vi "getSub2dArray.vi"(9 "Idx of Raw 1":i32[](array[numeric]), 10 "Idx of Raw 0":i32[](array[numeric]), 11 "2D Array":dbl[][](array[numeric])) -> (3 "Sub-Array":dbl[][](array[numeric]))   [LabVIEW 2016]
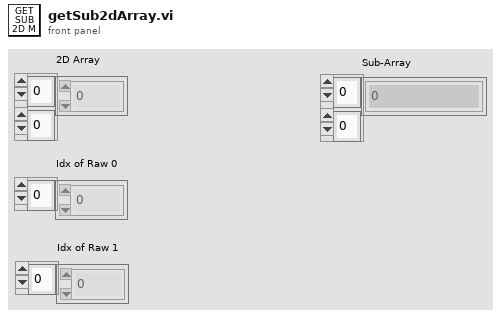
[diagram p1: front panel]
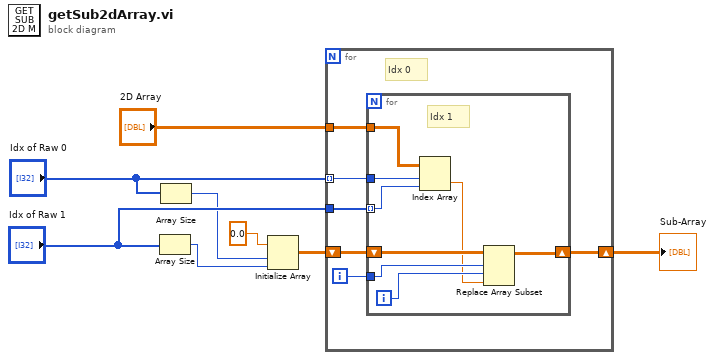
[diagram p0: block diagram]
diagram:
  n1 = Array Size(array="Idx of Raw 1") -> (size(s)=w2:i32)
  n2 = Array Size(array="Idx of Raw 0") -> (size(s)=w3:i32)
  n3 = Initialize Array(0.0 ("element"), w3, w2) -> (w6:dbl[][])
  n4 = for {
    shift-right: [w10] -> w1
    shift-left: w6 -> [w11]
    tunnel: "Idx of Raw 0" -> [w14] mode=indexing
    tunnel: "Idx of Raw 1" -> [w13]
    tunnel: "2D Array" -> [w12]
    i -> [w9]
    # "Idx 0"
    n5 = for {
      shift-right: [w18] -> w10
      shift-left: w11 -> [w19]
      tunnel: w14 -> [w21]
      tunnel: w13 -> [w20] mode=indexing
      tunnel: w12 -> [w22]
      tunnel: w9 -> [w17]
      i -> [w16]
      # "Idx 1"
      n6 = Index Array(array=w22, index (row)=w21, index (col)=w20) -> (element=w15:dbl)
      n7 = Replace Array Subset(array=w19, new element=w15, index (row)=w17, index (col)=w16) -> (w18:dbl[][])
    }
  }
  "Sub-Array" <- w1
